vi "dfd_Halfband Filter Design Equiripple TF Modify.vi"(8 "error in (no error)":errorcluster, 11 "h in":dbl[](array[numeric])) -> (0 "error out":errorcluster, 2 "order out":i32, 3 "h out":dbl[](array[numeric]))   [LabVIEW 2017, in "NI_DigFilter_Process.lvlib"]
uses:
  <vilib>/addons/Digital Filter Design/NI_DigFilter_Process.lvlib
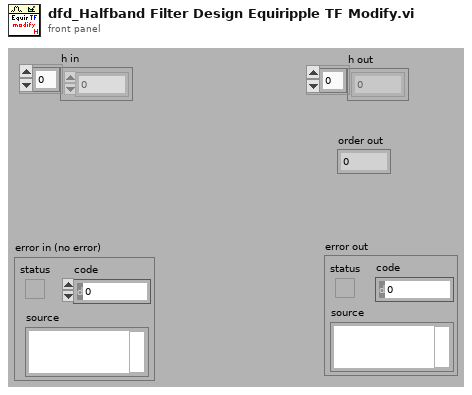
[diagram p1: front panel]
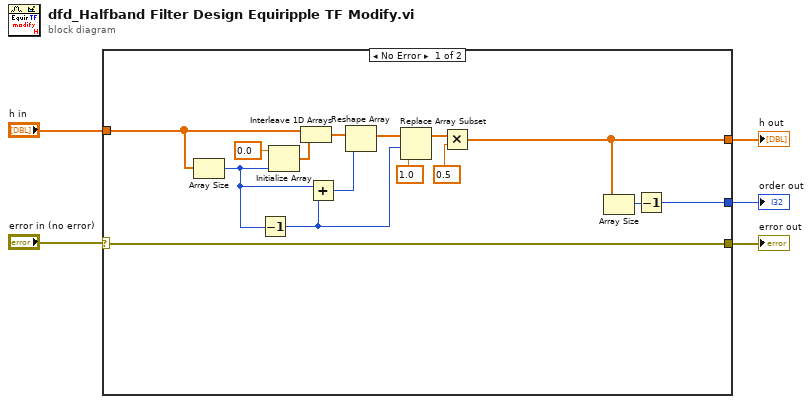
[diagram p0: block diagram]
diagram:
  n1 = case shown="No Error" "error in (no error)" {
    selector: "error in (no error)" -> [w7 w21]
    tunnel: "h in" -> [w8 _]
    tunnel: [w9 _] -> w3
    tunnel: [w7 w21] -> w2
    tunnel: [w6 _] -> w1
    frame No Error {
      n2 = Array Size(array=w8) -> (size(s)=w13:i32)
      n3 = Decrement(x=w13) -> (x-1=w12:i32)
      n4 = Initialize Array(0.0 ("element"), w13) -> (w19:dbl[])
      n5 = Interleave 1D Arrays(w8, w19) -> (w10:dbl[])
      n6 = Add(x=w13, y=w12) -> (x+y=w11:i32)
      n7 = Reshape Array(w10, w11) -> (w18:dbl[])
      n8 = Replace Array Subset(array=w18, new element=1.0 ("new element/subarray"), index=w12) -> (w16:dbl[])
      n9 = Multiply(x=w16, y=0.5 ("new element/subarray")) -> (x*y=w6:dbl[])
      n10 = Array Size(array=w6) -> (size(s)=w20:i32)
      n11 = Decrement(x=w20) -> (x-1=w9:i32)
    }
    frame Error {
    }
  }
  "order out" <- w3
  "error out" <- w2
  "h out" <- w1
